vi "Export matches to CSV.vi"(6 "Score":sgl[](array[numeric]), 7 "append to file? (T)":bool=TRUE, 8 "PosY":sgl[](array[numeric]), 9 "PosX":sgl[](array[numeric]), 10 "filenames for processing":string[](array[string]), 11 "Data Export Filepath":path) -> ()   [LabVIEW 2012]
uses:
  <vilib>/Utility/file.llb/Write To Spreadsheet File (string).vi
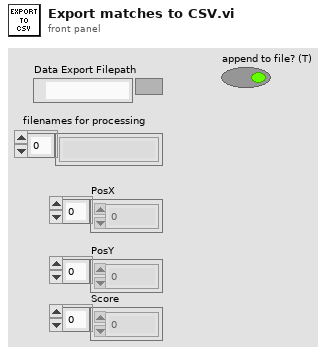
[diagram p1: front panel]
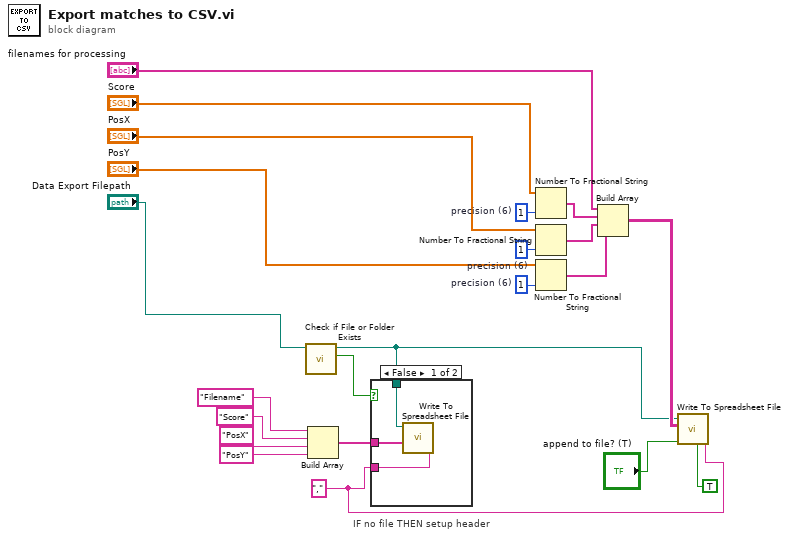
[diagram p0: block diagram]
diagram:
  w20 = "," ("delimiter (\\t)")
  w10 = i16 1  # precision (6)
  w11 = i16 1  # precision (6)
  w12 = i16 1  # precision (6)
  n1 = call <vilib>:"Check if File or Folder Exists.vi"("path"="Data Export Filepath") -> ("file or folder exists?"=w2:bool, "dup path"=w1:path)  [unwired: 8 in, 1 out]
  n2 = Build Array("Filename", "Score", "PosX", "PosY") -> (w18:string[])
  n3 = case "IF no file THEN setup header" shown="False" w2 {
    tunnel: w20 -> [w25 _]
    tunnel: w18 -> [w24 _]
    tunnel: w1 -> [w23 _]
    frame False {
      n4 = call-poly <vilib>:"Write To Spreadsheet File.vi"("delimiter (\\t)"=w25, "1D data"=w24, "file path (dialog if empty)"=w23) -> ()  [unwired: 5 in, 1 out]
    }
    frame True {
    }
  }
  n5 = Number To Fractional String(number="Score", precision (6)=w12) -> (F-format string=w9:string[])  [unwired: 2 in]
  n6 = Number To Fractional String(number="PosX", precision (6)=w11) -> (F-format string=w13:string[])  [unwired: 2 in]
  n7 = Number To Fractional String(number="PosY", precision (6)=w10) -> (F-format string=w21:string[])  [unwired: 2 in]
  n8 = Build Array("filenames for processing", w9, w13, w21) -> (w22:string[][])
  n9 = call-poly <vilib>:"Write To Spreadsheet File.vi"("delimiter (\\t)"=w20, "transpose? (no:F)"=TRUE, "append to file? (new file:F)"="append to file? (T)", "2D data"=w22, "file path (dialog if empty)"=w1) -> ()  [unwired: 3 in, 1 out]
